vi "Pre Launch Init.vi"(11 "SpectroscopyUI in":refnum<class "SpectroscopyUI.lvclass">) -> (0 "error out":errorcluster, 3 "SpectroscopyUI out":refnum<class "SpectroscopyUI.lvclass">)   [LabVIEW 2023, in "SpectroscopyUI.lvlib" / "SpectroscopyUI.lvclass"]
doc: "(<B>Filename</B>: Actor Framework.lvlib:Actor.lvclass:Pre Launch Init.vi)\n\nDefines behavior that occurs after the Launch Nested Actor method is invoked but before the actor's Actor Core method begins running.\n\nBy default, this method does nothing. A descendant class may override it to define behavior."
uses:
  SpectroscopyUI.lvclass
  <vilib>/ActorFramework/Actor/Actor.lvclass
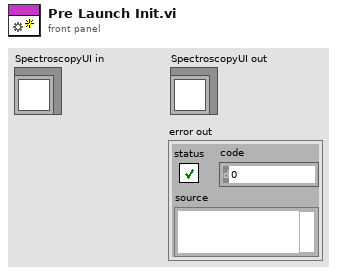
[diagram p1: front panel]
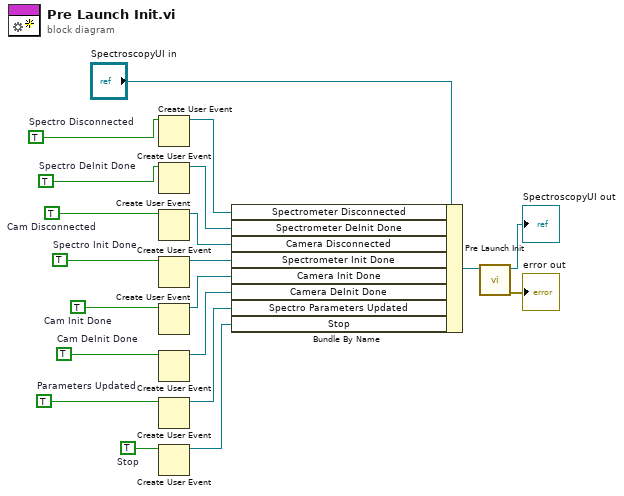
[diagram p0: block diagram]
diagram:
  w6 = TRUE  # Cam DeInit Done
  w7 = TRUE  # Spectro Init Done
  w10 = TRUE  # Spectro DeInit Done
  w9 = TRUE  # Spectro Disconnected
  w8 = TRUE  # Cam Disconnected
  w14 = TRUE  # Parameters Updated
  w15 = TRUE  # Cam Init Done
  w18 = TRUE  # Stop
  n1 = Create User Event(user event datatype=w9) -> (user event=w5:refnum<user-event>)  [unwired: 1 in, 1 out]
  n2 = Create User Event(user event datatype=w10) -> (user event=w4:refnum<user-event>)  [unwired: 1 in, 1 out]
  n3 = Create User Event(user event datatype=w8) -> (user event=w3:refnum<user-event>)  [unwired: 1 in, 1 out]
  n4 = Create User Event(user event datatype=w7) -> (user event=w1:refnum<user-event>)  [unwired: 1 in, 1 out]
  n5 = Create User Event(user event datatype=w15) -> (user event=w11:refnum<user-event>)  [unwired: 1 in, 1 out]
  n6 = Create User Event(user event datatype=w6) -> (user event=w2:refnum<user-event>)  [unwired: 1 in, 1 out]
  n7 = Create User Event(user event datatype=w14) -> (user event=w12:refnum<user-event>)  [unwired: 1 in, 1 out]
  n8 = Create User Event(user event datatype=w18) -> (user event=w13:refnum<user-event>)  [unwired: 1 in, 1 out]
  n9 = Bundle By Name(cluster="SpectroscopyUI in", "Spectrometer Disconnected"=w5, "Spectrometer DeInit Done"=w4, "Camera Disconnected"=w3, "Spectrometer Init Done"=w1, "Camera Init Done"=w11, "Camera DeInit Done"=w2, "Spectro Parameters Updated"=w12, "Stop"=w13) -> (w16:refnum<class "SpectroscopyUI.lvclass">)
  n10 = call-parent "Pre Launch Init.vi"("Actor in"=w16) -> ("error out"=→"error out":errorcluster, "Actor out"=→"SpectroscopyUI out":refnum<class "SpectroscopyUI.lvclass">)  [unwired: 9 in]
